vi "Forward Kinematics.vi"(11 "joints":dbl[](array[numeric])) -> (2 "exist":bool, 3 "p":dbl[](array[numeric]))   [LabVIEW 2013]
uses:
  <vilib>/Analysis/baseanly.llb/A x Vector.vi
  <vilib>/Analysis/_algsub.llb/Real Vector Norm.vi
  <vilib>/Analysis/baseanly.llb/Outer Product.vi
  <vilib>/Analysis/baseanly.llb/Real Outer Product.vi
  <vilib>/robotics/Kinematics/Create Lie Group Matrix.vi
  <vilib>/Analysis/7linalg.llb/Create Special Matrix.vi
  <vilib>/Analysis/7linalg.llb/Create Special Real Matrix.vi
  <vilib>/Analysis/Matrix/Numeric/Multiply/Multiply.vi
  <vilib>/Analysis/Matrix/Numeric/Multiply/Multiply - RM,R.vi
  <vilib>/Analysis/Matrix/Numeric/Multiply/Multiply - R,RM.vi
  <vilib>/Analysis/Matrix/Numeric/Add/Add.vi
  <vilib>/Analysis/Matrix/Numeric/Add/Add - RM,RM.vi
  <vilib>/robotics/Kinematics/NI_Kinematics.lvlib
  <vilib>/Analysis/NI_AALBase.lvlib
  <vilib>/Analysis/NI_AALPro.lvlib
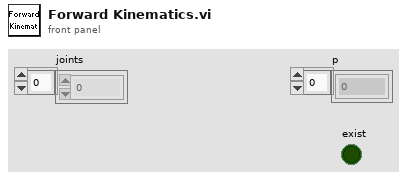
[diagram p1: front panel]
types:
  T1 = typedef "NI_Matrix.lvlib/RealMatrix.ctl" = dbl[][]
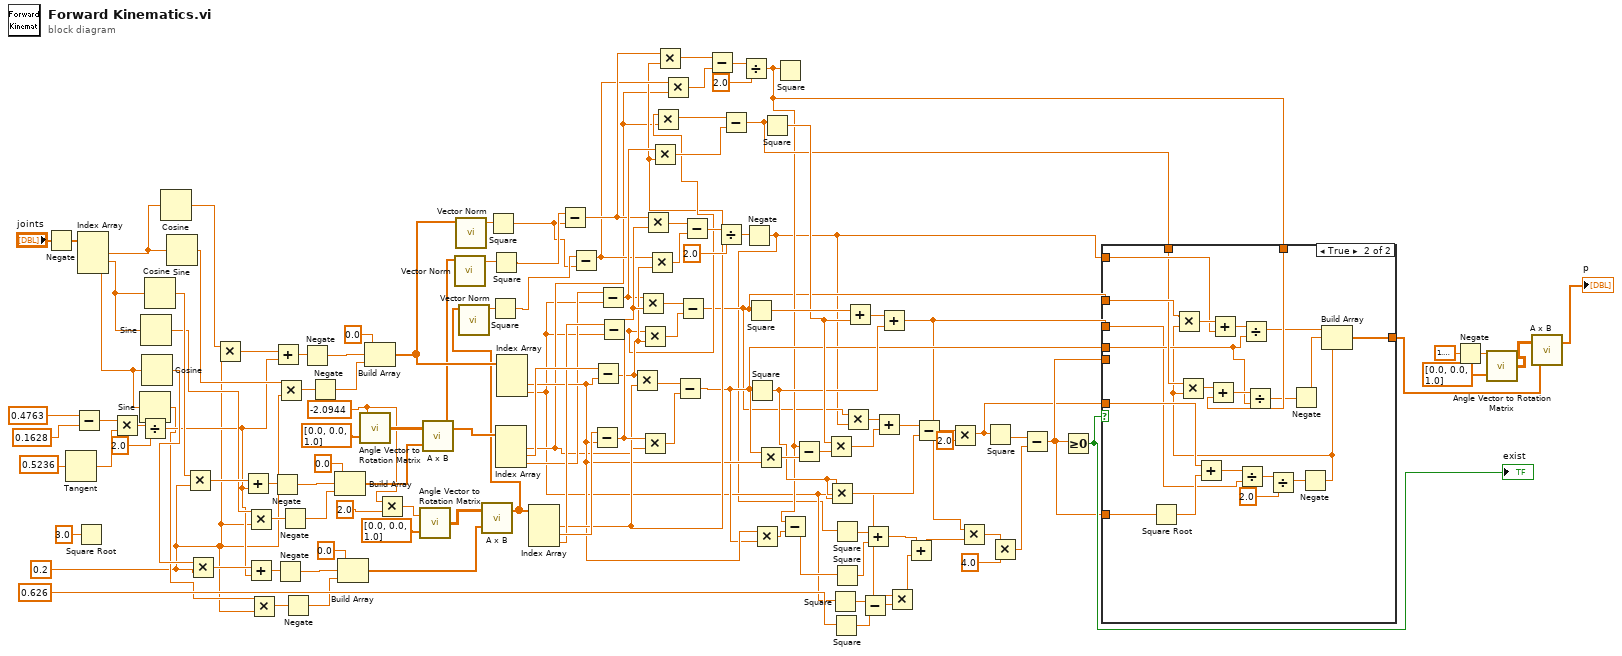
[diagram p0: block diagram]
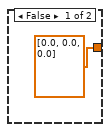
[diagram p2: hidden frame]
diagram:
  w17 = -2.0944
  w24 = 0.2 ("rf")
  n1 = Negate(x="joints") -> (-x=w20:dbl[])
  n2 = Tangent(1:0.5236 ("x")) -> (0:w123:dbl)
  n3 = Subtract(x=0.4763 ("f"), y=0.1628 ("e")) -> (x-y=w124:dbl)
  n4 = Square Root(x=3.0) -> ()  [unwired: 1 out]
  n5 = Index Array(array=w20) -> (element #1=w117:dbl, element #2=w43:dbl, element #3=w42:dbl)  [unwired: 3 in]
  n6 = Multiply(x=w124, y=w123) -> (x*y=w122:dbl)
  n7 = Sine(x=w42) -> (sin(x)=w25:dbl)
  n8 = Divide(x=w122, y=2.0) -> (x/y=w26:dbl)
  n9 = Sine(x=w43) -> (sin(x)=w27:dbl)
  n10 = Cosine(x=w42) -> (cos(x)=w28:dbl)
  n11 = Cosine(x=w43) -> (cos(x)=w29:dbl)
  n12 = Cosine(x=w117) -> (cos(x)=w120:dbl)
  n13 = Sine(x=w117) -> (sin(x)=w116:dbl)
  n14 = Multiply(x=w29, y=w24) -> (x*y=w41:dbl)
  n15 = Multiply(x=w28, y=w24) -> (x*y=w30:dbl)
  n16 = Multiply(x=w120, y=w24) -> (x*y=w119:dbl)
  n17 = Add(x=w41, y=w26) -> (x+y=w40:dbl)
  n18 = Multiply(x=w27, y=w24) -> (x*y=w39:dbl)
  n19 = Add(x=w30, y=w26) -> (x+y=w31:dbl)
  n20 = Multiply(x=w25, y=w24) -> (x*y=w32:dbl)
  n21 = Negate(x=w40) -> (-x=w38:dbl)
  n22 = Add(x=w119, y=w26) -> (x+y=w118:dbl)
  n23 = Negate(x=w31) -> (-x=w33:dbl)
  n24 = Multiply(x=w116, y=w24) -> (x*y=w115:dbl)
  n25 = Negate(x=w39) -> (-x=w37:dbl)
  n26 = Negate(x=w32) -> (-x=w34:dbl)
  n27 = Negate(x=w118) -> (-x=w114:dbl)
  n28 = Negate(x=w115) -> (-x=w113:dbl)
  n29 = Build Array(0.0 ("element"), w38, w37) -> (w23:dbl[])
  n30 = Build Array(0.0 ("element"), w33, w34) -> (w22:dbl[])
  n31 = call <vilib>:"Angle Vector to Rotation Matrix.vi"("vector"=dbl[] [0.0, 0.0, 1.0], "angle"=w17) -> ("rotation matrix"=w110:T1)
  n32 = Build Array(0.0 ("element"), w114, w113) -> (w105:dbl[])
  n33 = Multiply(x=w17, y=2.0) -> (x*y=w15:dbl)
  n34 = call <vilib>:"Angle Vector to Rotation Matrix.vi"("vector"=dbl[] [0.0, 0.0, 1.0], "angle"=w15) -> ("rotation matrix"=w18:T1)
  n35 = call-poly <vilib>:"A x B.vi"("Vector"=w23, "A"=w110) -> ("A x Vector"=w104:dbl[])  [unwired: 1 out]
  n36 = call-poly <vilib>:"Vector Norm.vi"("Input Vector"=w104) -> ("norm"=w12:dbl)  [unwired: 9 in, 1 out]
  n37 = call-poly <vilib>:"Vector Norm.vi"("Input Vector"=w105) -> ("norm"=w10:dbl)  [unwired: 9 in, 1 out]
  n38 = call-poly <vilib>:"A x B.vi"("Vector"=w22, "A"=w18) -> ("A x Vector"=w103:dbl[])  [unwired: 1 out]
  n39 = call-poly <vilib>:"Vector Norm.vi"("Input Vector"=w103) -> ("norm"=w14:dbl)  [unwired: 9 in, 1 out]
  n40 = Square(x=w10) -> (x^2=w9:dbl)
  n41 = Square(x=w14) -> (x^2=w13:dbl)
  n42 = Square(x=w12) -> (x^2=w11:dbl)
  n43 = Index Array(array=w104) -> (element #1=w7:dbl, element #2=w109:dbl, element #3=w8:dbl)  [unwired: 3 in]
  n44 = Index Array(array=w105) -> (element #2=w71:dbl, element #3=w6:dbl)  [unwired: 3 in, 1 out]
  n45 = Index Array(array=w103) -> (element #1=w86:dbl, element #2=w107:dbl, element #3=w101:dbl)  [unwired: 3 in]
  n46 = Subtract(x=w11, y=w9) -> (x-y=w89:dbl)
  n47 = Subtract(x=w13, y=w9) -> (x-y=w87:dbl)
  n48 = Subtract(x=w107, y=w71) -> (x-y=w99:dbl)
  n49 = Subtract(x=w109, y=w71) -> (x-y=w98:dbl)
  n50 = Subtract(x=w8, y=w6) -> (x-y=w92:dbl)
  n51 = Subtract(x=w101, y=w6) -> (x-y=w88:dbl)
  n52 = Multiply(x=w98, y=w86) -> (x*y=w108:dbl)
  n53 = Multiply(x=w92, y=w99) -> (x*y=w102:dbl)
  n54 = Multiply(x=w88, y=w98) -> (x*y=w100:dbl)
  n55 = Multiply(x=w99, y=w7) -> (x*y=w106:dbl)
  n56 = Multiply(x=w89, y=w99) -> (x*y=w97:dbl)
  n57 = Multiply(x=w87, y=w98) -> (x*y=w96:dbl)
  n58 = Multiply(x=w92, y=w86) -> (x*y=w90:dbl)
  n59 = Multiply(x=w88, y=w7) -> (x*y=w91:dbl)
  n60 = Multiply(x=w89, y=w86) -> (x*y=w85:dbl)
  n61 = Multiply(x=w87, y=w7) -> (x*y=w84:dbl)
  n62 = Subtract(x=w108, y=w106) -> (x-y=w53:dbl)
  n63 = Subtract(x=w102, y=w100) -> (x-y=w5:dbl)
  n64 = Subtract(x=w97, y=w96) -> (x-y=w95:dbl)
  n65 = Subtract(x=w85, y=w84) -> (x-y=w83:dbl)
  n66 = Divide(x=w95, y=2.0) -> (x/y=w93:dbl)
  n67 = Subtract(x=w91, y=w90) -> (x-y=w52:dbl)
  n68 = Divide(x=w83, y=2.0) -> (x/y=w51:dbl)
  n69 = Negate(x=w93) -> (-x=w4:dbl)
  n70 = Square(x=w5) -> (x^2=w81:dbl)
  n71 = Square(x=w53) -> (x^2=w62:dbl)
  n72 = Multiply(x=w71, y=w53) -> (x*y=w70:dbl)
  n73 = Multiply(x=w53, y=w71) -> (x*y=w79:dbl)
  n74 = Square(x=w52) -> (x^2=w77:dbl)
  n75 = Square(x=w51) -> ()  [unwired: 1 out]
  n76 = Subtract(x=w51, y=w70) -> (x-y=w69:dbl)
  n77 = Subtract(x=w51, y=w79) -> (x-y=w78:dbl)
  n78 = Multiply(x=w77, y=w78) -> (x*y=w76:dbl)
  n79 = Multiply(x=w62, y=w6) -> (x*y=w74:dbl)
  n80 = Square(x=w6) -> (x^2=w66:dbl)
  n81 = Square(x=0.626 ("re")) -> (x^2=w64:dbl)
  n82 = Square(x=w4) -> (x^2=w68:dbl)
  n83 = Square(x=w69) -> (x^2=w67:dbl)
  n84 = Multiply(x=w5, y=w4) -> (x*y=w3:dbl)
  n85 = Add(x=w81, y=w77) -> (x+y=w80:dbl)
  n86 = Subtract(x=w66, y=w64) -> (x-y=w63:dbl)
  n87 = Add(x=w68, y=w67) -> (x+y=w61:dbl)
  n88 = Add(x=w3, y=w76) -> (x+y=w75:dbl)
  n89 = Add(x=w80, y=w62) -> (x+y=w48:dbl)
  n90 = Multiply(x=w62, y=w63) -> (x*y=w60:dbl)
  n91 = Add(x=w61, y=w60) -> (x+y=w59:dbl)
  n92 = Subtract(x=w75, y=w74) -> (x-y=w73:dbl)
  n93 = Multiply(x=w73, y=2.0) -> (x*y=w49:dbl)
  n94 = Multiply(x=w48, y=w59) -> (x*y=w58:dbl)
  n95 = Square(x=w49) -> (x^2=w56:dbl)
  n96 = Multiply(x=w58, y=4.0) -> (x*y=w55:dbl)
  n97 = Subtract(x=w56, y=w55) -> (x-y=w50:dbl)
  n98 = Greater Or Equal To 0?(x=w50) -> (x >= 0?=w54:bool)
  "exist" <- w54
  n99 = case shown="True" w54 {
    tunnel: w50 -> [_ _]
    tunnel: w5 -> [_ w151]
    tunnel: w4 -> [_ w149]
    tunnel: w53 -> [_ w143]
    tunnel: w52 -> [_ w147]
    tunnel: w51 -> [_ w145]
    tunnel: w50 -> [_ w142]
    tunnel: w49 -> [_ w140]
    tunnel: w48 -> [_ w138]
    tunnel: [dbl[] [0.0, 0.0, 0.0] w135] -> w45
    frame False {
    }
    frame True {
      n100 = Square Root(x=w142) -> (sqrt(x)=w141:dbl)
      n101 = Add(x=w140, y=w141) -> (x+y=w139:dbl)
      n102 = Divide(x=w139, y=w138) -> (x/y=w137:dbl)
      n103 = Divide(x=w137, y=2.0) -> (x/y=w134:dbl)
      n104 = Negate(x=w134) -> (-x=w133:dbl)
      n105 = Multiply(x=w151, y=w133) -> (x*y=w150:dbl)
      n106 = Multiply(x=w147, y=w133) -> (x*y=w146:dbl)
      n107 = Add(x=w146, y=w145) -> (x+y=w144:dbl)
      n108 = Add(x=w150, y=w149) -> (x+y=w148:dbl)
      n109 = Divide(x=w148, y=w143) -> (x/y=w132:dbl)
      n110 = Divide(x=w144, y=w143) -> (x/y=w131:dbl)
      n111 = Negate(x=w131) -> (-x=w130:dbl)
      n112 = Build Array(w132, w130, w133) -> (w135:dbl[])
    }
  }
  n113 = Negate(x=1.5707963267948966) -> (-x=w1:dbl)
  n114 = call <vilib>:"Angle Vector to Rotation Matrix.vi"("vector"=dbl[] [0.0, 0.0, 1.0], "angle"=w1) -> ("rotation matrix"=w46:T1)
  n115 = call-poly <vilib>:"A x B.vi"("Vector"=w45, "A"=w46) -> ("A x Vector"=→"p":dbl[])  [unwired: 1 out]
